vi "(Test) Power Control.vi"() -> ()   [LabVIEW 2017]
uses:
  Controls/(Ctrl) System State.ctl
  Controls/(Ctrl) State_HVPS CMD.ctl
  Controls/(Ctrl) State_Parcing.ctl
panel:
  in  "ADC Read":bool
  in  "Set mA":dbl
  in  "mA SET":bool
  in  "Set V":dbl
  in  "V SET":bool
  in  "KV Read":bool
  out "V":dbl
  out "G1 System State":T1
  out "mA":dbl
  in  "mA Read":bool
  out "Operation Mode":string
  out "HV State":string
  out "System State":string
  in  "State Read":bool
  in  "Power OFF":bool
  in  "Power ON":bool
  in  "정지":bool
  # "Group.1"
  # "Voltage Mode On"
  # "Current Mode On"
  # "HV On"
  # "Regulator Error"
  # "Local Mode"
  # "System Fault"
  # "Adjustable Overload Fault"
  # "Over Temperature"
  # "Arc Fault"
  # "Over Power"
  # "Over Current"
  # "Over Voltage Fault"
  # "HV Inhibited"
  # "Interlock open"
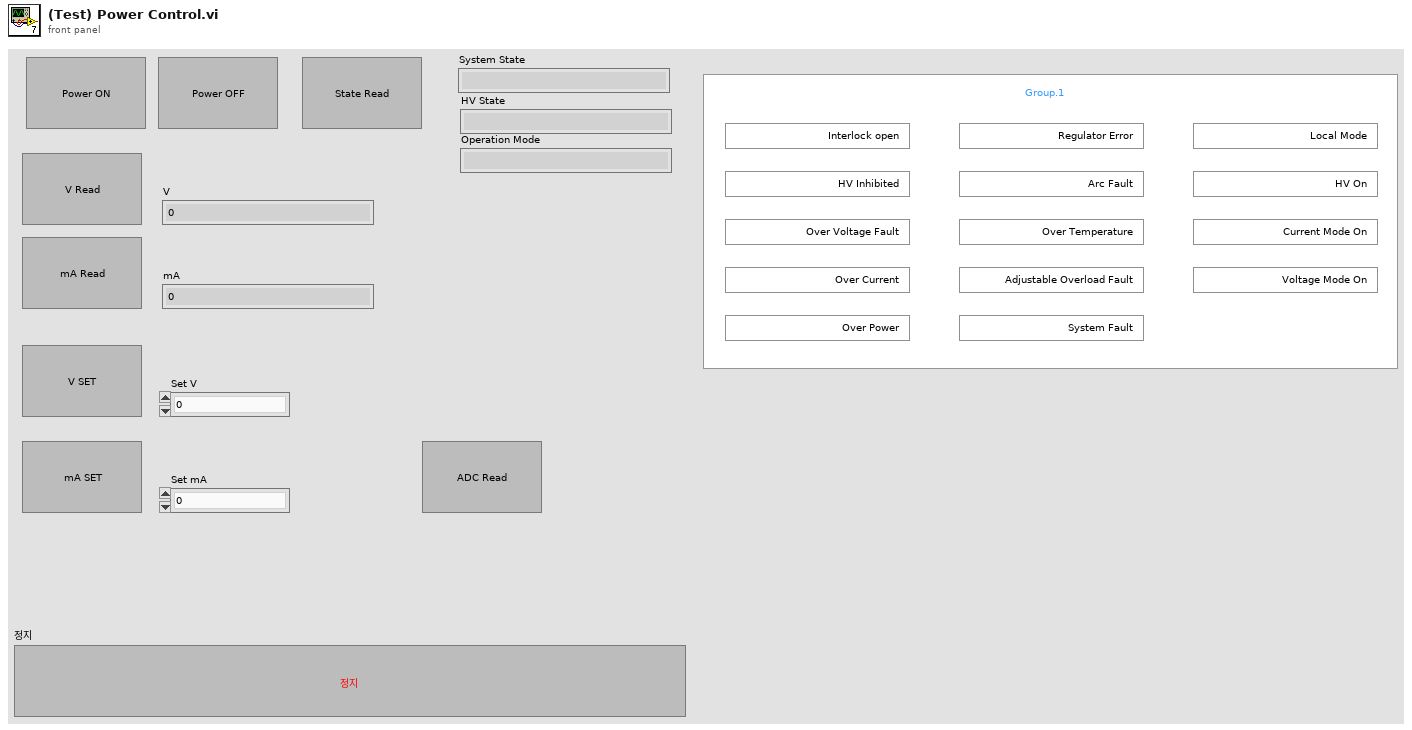
[diagram p1: front panel]
types:
  T1 = typedef "(Ctrl) System State.ctl" = cluster{"Interlock open":bool, "HV Inhibited":bool, "Over Voltage Fault":bool, "Over Current":bool, "Over Power":bool, "Regulator Error":bool, "Arc Fault":bool, "Over Temperature":bool, "Adjustable Overload Fault":bool, "System Fault":bool, "Remote Mode":bool, "HV On":bool, "Current Mode On":bool, "Voltage Mode On":bool}
  T2 = typedef "(Ctrl) State_HVPS CMD.ctl" = enum16{"Open", "Rx : V", "Rx : mA", "Rx : State", "Rx : ADC", "Tx : Set V", "Tx : Set mA", "Tx : ON", "Tx : OFF", "Close"}
  T3 = typedef "(Ctrl) State_Parcing.ctl" = enum16{"Default", "Set V", "Set mA", "Get V", "Get mA", "Get ADC"}
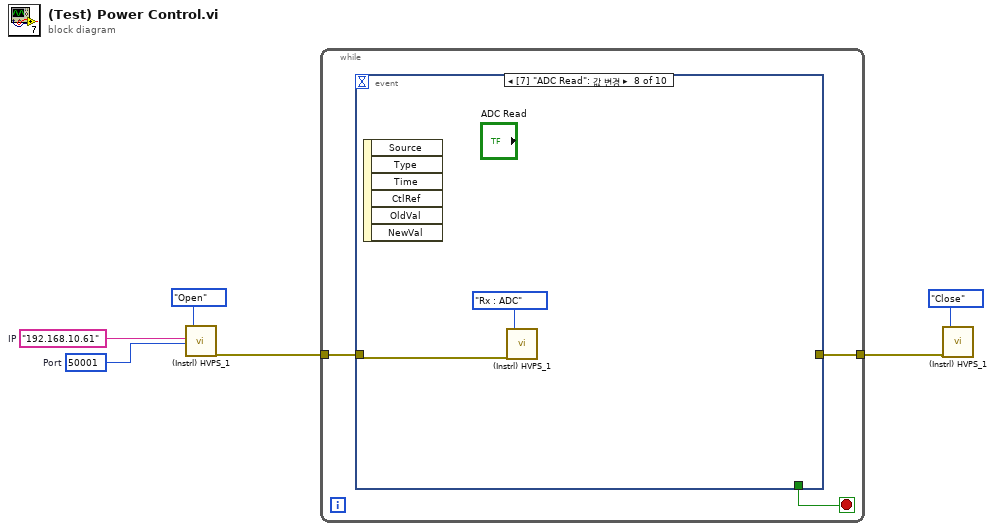
[diagram p0: block diagram]
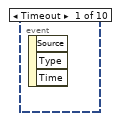
[diagram p2: hidden frame]
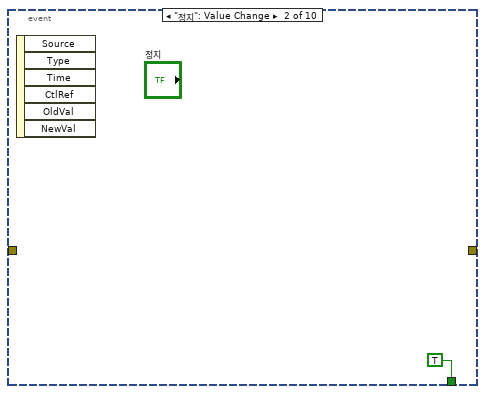
[diagram p3: hidden frame]
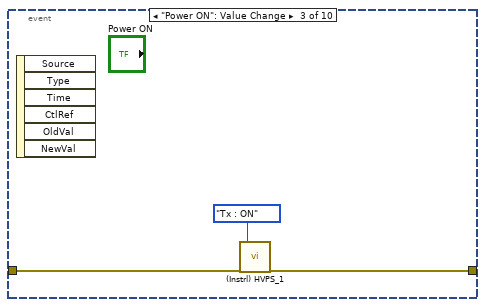
[diagram p4: hidden frame]
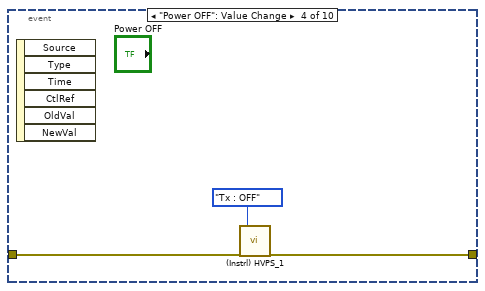
[diagram p5: hidden frame]
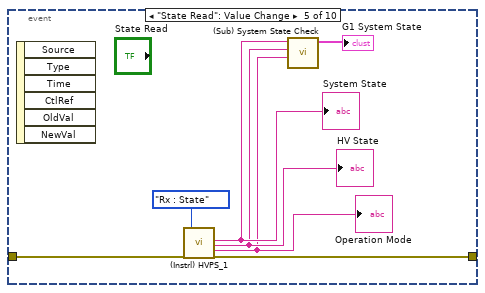
[diagram p6: hidden frame]
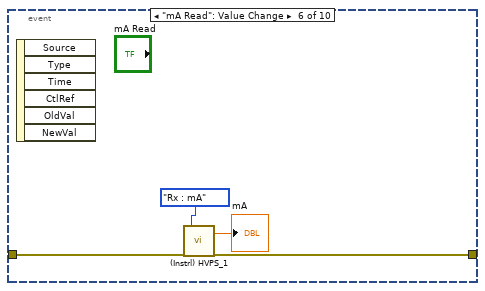
[diagram p7: hidden frame]
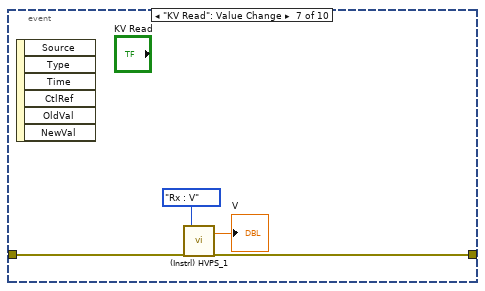
[diagram p8: hidden frame]
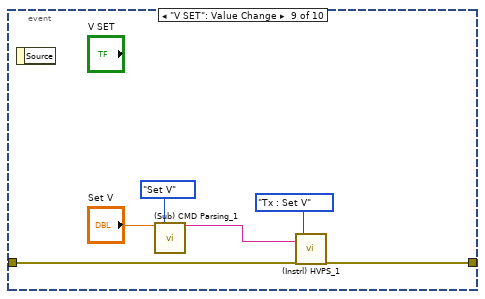
[diagram p9: hidden frame]
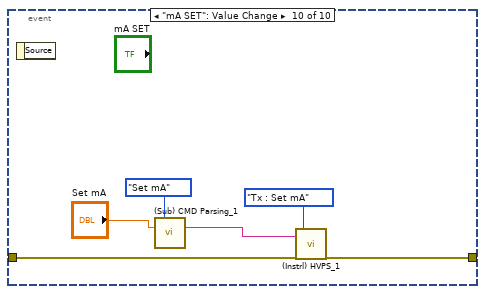
[diagram p10: hidden frame]
diagram:
  w4 = u16 50001  # Port
  w5 = "192.168.10.61"  # IP
  n1 = call "(Instrl) HVPS_1.vi"("IP"=w5, "Port"=w4, "CMD"=(Ctrl)_State_HVPS_CMD."Open" ("State")) -> ("error out"=w3:errorcluster)  [unwired: 11 in, 5 out]
  n2 = while {
    tunnel: w3 -> [w8]
    tunnel: [w7] -> w1
    stop <- w9 stop-if-true
    n3 = event shown="[7] \"ADC Read\": 값 변경" {
      selector: _ -> [_ _ _ _ _ _ _ _ _ _]
      dyn-events: _ -> [_ _ _ _ _ _ _ _ _ _]
      timeout: _ -> [_ _ _ _ _ _ _ _ _ _]
      tunnel: [_ TRUE _ _ _ _ _ _ _ _] -> w9
      tunnel: w8 -> [_ _ w12 w15 w22 w26 w30 w33 w39 w45]
      tunnel: [_ _ w11 w14 w21 w25 w29 _ w38 w44] -> w7
      event Timeout {
        n4 = event-data() -> ()  [unwired: 1 in, 3 out]
      }
      event "정지": Value Change {
        n5 = event-data() -> ()  [unwired: 1 in, 6 out]
      }
      event "Power ON": Value Change {
        n6 = event-data() -> ()  [unwired: 1 in, 6 out]
        n7 = call "(Instrl) HVPS_1.vi"("error in (no error)"=w12, "CMD"=(Ctrl)_State_HVPS_CMD."Tx : ON" ("State")) -> ("error out"=w11:errorcluster)  [unwired: 12 in, 5 out]
      }
      event "Power OFF": Value Change {
        n8 = event-data() -> ()  [unwired: 1 in, 6 out]
        n9 = call "(Instrl) HVPS_1.vi"("error in (no error)"=w15, "CMD"=(Ctrl)_State_HVPS_CMD."Tx : OFF" ("State")) -> ("error out"=w14:errorcluster)  [unwired: 12 in, 5 out]
      }
      event "State Read": Value Change {
        n10 = event-data() -> ()  [unwired: 1 in, 6 out]
        n11 = call "(Instrl) HVPS_1.vi"("error in (no error)"=w22, "CMD"=(Ctrl)_State_HVPS_CMD."Rx : State" ("State")) -> ("System State"=w20:string, "HV State"=w19:string, "Operation Mode"=w18:string, "error out"=w21:errorcluster)  [unwired: 12 in, 2 out]
        "System State" <- w20
        "HV State" <- w19
        "Operation Mode" <- w18
        n12 = call "(Sub) System State Check.vi"("Read  Mode"=w18, "Read HV State"=w19, "Read System State"=w20) -> ("Out System State"=→"G1 System State":T1)  [unwired: 6 in, 2 out]
      }
      event "mA Read": Value Change {
        n13 = event-data() -> ()  [unwired: 1 in, 6 out]
        n14 = call "(Instrl) HVPS_1.vi"("error in (no error)"=w26, "CMD"=(Ctrl)_State_HVPS_CMD."Rx : mA" ("State")) -> ("Get mA"=→"mA":dbl, "error out"=w25:errorcluster)  [unwired: 12 in, 4 out]
      }
      event "KV Read": Value Change {
        n15 = event-data() -> ()  [unwired: 1 in, 6 out]
        n16 = call "(Instrl) HVPS_1.vi"("error in (no error)"=w30, "CMD"=(Ctrl)_State_HVPS_CMD."Rx : V" ("State")) -> ("Get mA"=→"V":dbl, "error out"=w29:errorcluster)  [unwired: 12 in, 4 out]
      }
      event "ADC Read": Value Change {
        n17 = event-data() -> ()  [unwired: 1 in, 6 out]
        n18 = call "(Instrl) HVPS_1.vi"("error in (no error)"=w33, "CMD"=(Ctrl)_State_HVPS_CMD."Rx : ADC" ("State")) -> ()  [unwired: 12 in, 6 out]
      }
      event "V SET": Value Change {
        n19 = event-data() -> ()  [unwired: 1 in, 1 out]
        n20 = call "(Sub) CMD Parsing_1.vi"("Set V"="Set V", "State"=(Ctrl)_State_Parcing."Set V") -> ("CMD Set V"=w36:string)  [unwired: 9 in, 4 out]
        n21 = call "(Instrl) HVPS_1.vi"("Write Data"=w36, "error in (no error)"=w39, "CMD"=(Ctrl)_State_HVPS_CMD."Tx : Set V" ("State")) -> ("error out"=w38:errorcluster)  [unwired: 11 in, 5 out]
      }
      event "mA SET": Value Change {
        n22 = event-data() -> ()  [unwired: 1 in, 1 out]
        n23 = call "(Sub) CMD Parsing_1.vi"("State"=(Ctrl)_State_Parcing."Set mA", "Set mA"="Set mA") -> ("CMD Set mA"=w42:string)  [unwired: 9 in, 4 out]
        n24 = call "(Instrl) HVPS_1.vi"("Write Data"=w42, "error in (no error)"=w45, "CMD"=(Ctrl)_State_HVPS_CMD."Tx : Set mA" ("State")) -> ("error out"=w44:errorcluster)  [unwired: 11 in, 5 out]
      }
    }
  }
  n25 = call "(Instrl) HVPS_1.vi"("error in (no error)"=w1, "CMD"=(Ctrl)_State_HVPS_CMD."Close" ("State")) -> ()  [unwired: 12 in, 6 out]
